vi "getCurrentVersion.vi"(8 "error in (no error)":errorcluster, 11 "repoHandler in":refnum<class "repoHandler.lvclass">) -> (0 "error out":errorcluster, 1 "Log":string, 3 "repoHandler out":refnum<class "repoHandler.lvclass">, 4 "Local Version":string)   [LabVIEW 2013, in "repoHandler.lvclass"]
uses:
  repoHandler.lvclass
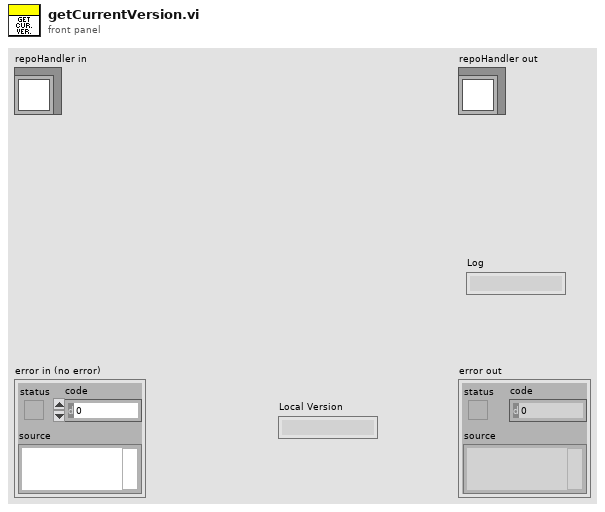
[diagram p1: front panel]
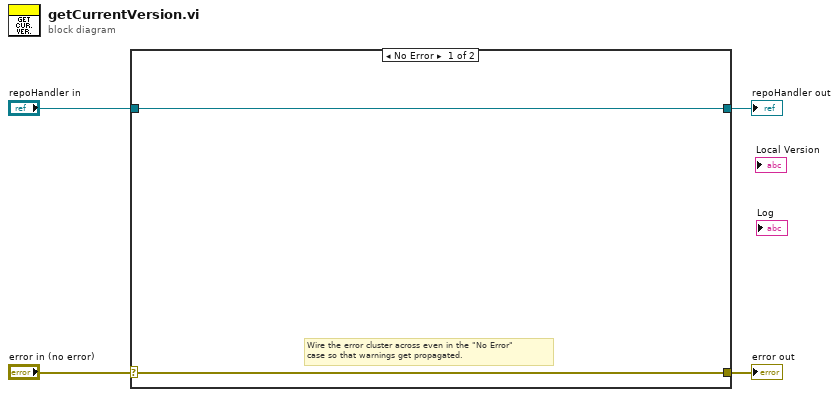
[diagram p0: block diagram]
diagram:
  n1 = case shown="No Error" "error in (no error)" {
    selector: "error in (no error)" -> [w5 w8]
    tunnel: [w5 w8] -> w3
    tunnel: [w6 w7] -> w1
    tunnel: "repoHandler in" -> [w6 w7]
    frame No Error {
      # "Wire the error cluster across even in the \"No Error\"\ncase so that warnings get propagated."
    }
    frame Error {
    }
  }
  "error out" <- w3
  "repoHandler out" <- w1
